vi "Enable VIO.vi"(0 "instrument handle":refnum<k15>, 1 "Bus Number":i32, 11 "error in":errorcluster) -> (4 "instrument handle out":refnum<k15>, 15 "error out":errorcluster)   [LabVIEW 2018, in "MIPI RFFE API.lvlib"]
uses:
  MIPI RFFE API.lvlib
  <instrlib>/niDigital/niDigital.llb/niDigital Output Function.ctl
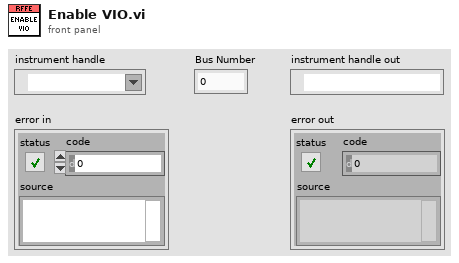
[diagram p1: front panel]
types:
  T1 = typedef "niDigital Output Function.ctl" = i32
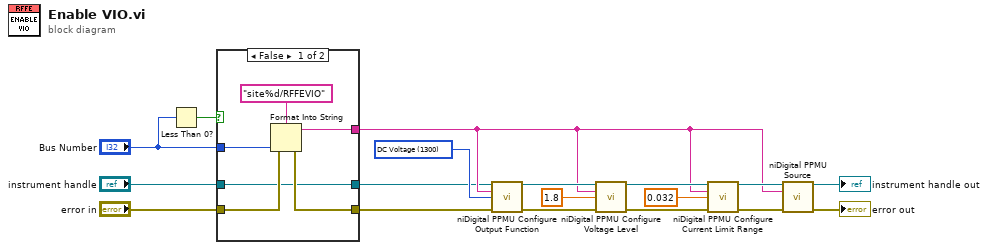
[diagram p0: block diagram]
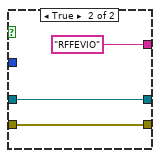
[diagram p2: hidden frame]
diagram:
  w13 = T1 1300 items=["DC Voltage"=1300, "DC Current"=1301] ("output function")
  n1 = Less Than 0?(x="Bus Number") -> (x < 0?=w4:bool)
  n2 = case shown="False" w4 {
    tunnel: "error in" -> [w21 w26]
    tunnel: [w22 "RFFEVIO" ("channel list")] -> w3
    tunnel: "Bus Number" -> [w23 _]
    tunnel: [w20 w26] -> w2
    tunnel: "instrument handle" -> [w19 w25]
    tunnel: [w19 w25] -> w1
    frame False {
      n3 = Format Into String(format string="site%d/RFFEVIO" ("channel list"), error in=w21, w23) -> (resulting string=w22:string, error out=w20:errorcluster)  [unwired: 1 in]
    }
    frame True {
    }
  }
  n4 = call <instrlib>:"niDigital PPMU Configure Output Function.vi"("instrument handle"=w1, "channel list"=w3, "output function"=w13, "error in"=w2) -> ("instrument handle out"=w12:refnum<k15>, "error out"=w11:errorcluster)  [unwired: 10 in]
  n5 = call <instrlib>:"niDigital PPMU Configure Voltage Level.vi"("instrument handle"=w12, "channel list"=w3, "voltage level (V)"=1.8, "error in"=w11) -> ("instrument handle out"=w7:refnum<k15>, "error out"=w9:errorcluster)  [unwired: 10 in]
  n6 = call <instrlib>:"niDigital PPMU Configure Current Limit Range.vi"("instrument handle"=w7, "channel list"=w3, "current limit range (A)"=0.032, "error in"=w9) -> ("instrument handle out"=w6:refnum<k15>, "error out"=w8:errorcluster)  [unwired: 10 in]
  n7 = call <instrlib>:"niDigital PPMU Source.vi"("instrument handle"=w6, "channel list"=w3, "error in"=w8) -> ("instrument handle out"=→"instrument handle out":refnum<k15>, "error out"=→"error out":errorcluster)  [unwired: 11 in]
